vi "Build2DParamArray.vi"(9 "Step Sizes":dbl[](array[numeric]), 10 "Final Values":dbl[](array[numeric]), 11 "Initial Values":dbl[](array[numeric])) -> (2 "Parameter Array":dbl[][](array[numeric]))   [LabVIEW 2013]
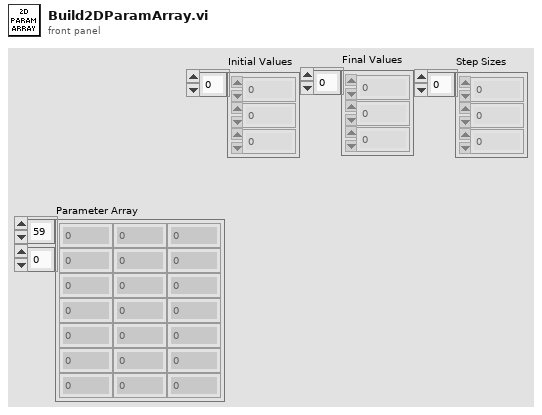
[diagram p1: front panel]
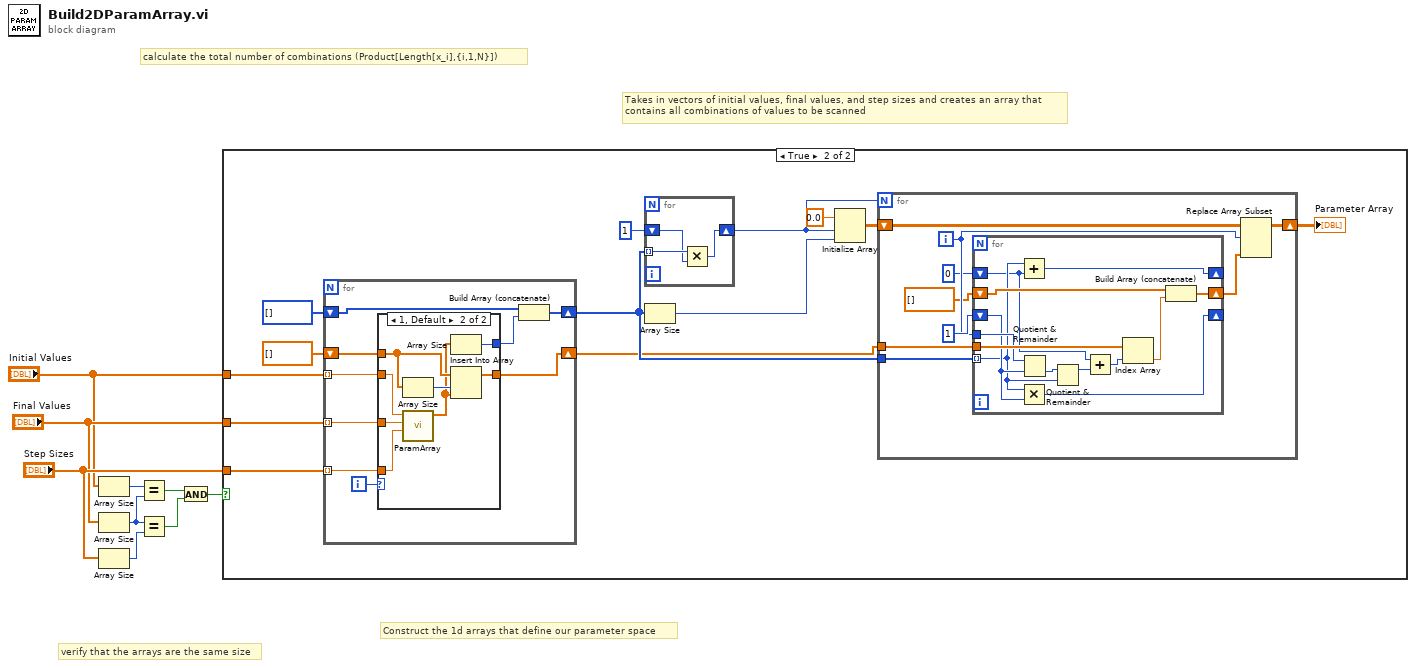
[diagram p0: block diagram]
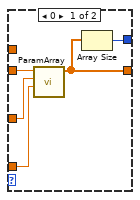
[diagram p3: hidden frame]
diagram:
  # "calculate the total number of combinations (Product[Length[x_i],{i,1,N}])"
  # "Construct the 1d arrays that define our parameter space"
  # "Takes in vectors of initial values, final values, and step sizes and creates an array that\ncontains all combinations of values to be scanned"
  # "verify that the arrays are the same size"
  n1 = Array Size(array="Initial Values") -> (size(s)=w7:i32)
  n2 = Array Size(array="Final Values") -> (size(s)=w8:i32)
  n3 = Array Size(array="Step Sizes") -> (size(s)=w9:i32)
  n4 = Equal?(x=w7, y=w8) -> (x = y?=w6:bool)
  n5 = Equal?(x=w8, y=w9) -> (x = y?=w5:bool)
  n6 = And(x=w6, y=w5) -> (x .and. y?=w4:bool)
  n7 = case shown="True" w4 {
    tunnel: "Step Sizes" -> [_ w22]
    tunnel: "Final Values" -> [_ w21]
    tunnel: "Initial Values" -> [_ w20]
    frame False {
    }
    frame True {
      n8 = for {
        tunnel: w22 -> [w56] mode=indexing
        tunnel: w21 -> [w55] mode=indexing
        tunnel: w20 -> [w54] mode=indexing
        shift-right: [w49] -> w13
        shift-left: dbl[] [] ("Array") -> [w48]
        shift-right: [w51] -> w14
        shift-left: i32[] [] -> [w52]
        i -> [w50]
        n9 = case shown="1, Default" w50 {
          tunnel: w56 -> [w61 w67]
          tunnel: w55 -> [w60 w68]
          tunnel: w54 -> [w59 w69]
          tunnel: [w57 w64] -> w49
          tunnel: [w58 w62] -> w53
          tunnel: w48 -> [_ w66]
          frame 0 {
            n10 = call "ParamArray.vi"("Step Size"=w61, "Final Value"=w60, "Initial Value"=w59) -> ("Array"=w57:dbl[])  [unwired: 8 in]
            n11 = Array Size(array=w57) -> (size(s)=w58:i32)
          }
          frame 1, Default {
            n12 = Array Size(array=w66) -> (size(s)=w65:i32)
            n13 = call "ParamArray.vi"("Step Size"=w67, "Final Value"=w68, "Initial Value"=w69) -> ("Array"=w63:dbl[])  [unwired: 8 in]
            n14 = Array Size(array=w63) -> (size(s)=w62:i32)
            n15 = Insert Into Array(array=w66, index=w65, new element=w63) -> (w64:dbl[])
          }
        }
        n16 = Build Array (concatenate)(w52, w53) -> (w51:i32[])
      }
      n17 = for {
        tunnel: w14 -> [w47] mode=indexing
        shift-right: [w46] -> w16
        shift-left: 1 -> [w45]
        n18 = Multiply(x=w47, y=w45) -> (x*y=w46:i32)
      }
      n19 = Array Size(array=w14) -> (size(s)=w19:i32)
      n20 = Initialize Array(0.0 ("element"), w16, w19) -> (w15:dbl[][])
      n21 = for {
        N: w16 -> [_]
        shift-right: [w30] -> w10
        shift-left: w15 -> [w31]
        tunnel: w14 -> [w29]
        tunnel: w13 -> [w27]
        i -> [w26]
        n22 = for {
          tunnel: w29 -> [w36] mode=indexing
          shift-right: [w44] -> _
          shift-left: 1 -> [w37]
          tunnel: w27 -> [w43]
          tunnel: w26 -> [w42]
          shift-right: [w38] -> w25
          shift-left: dbl[] [] -> [w39]
          shift-right: [w35] -> _
          shift-left: 0 -> [w34]
          n23 = Add(x=w36, y=w34) -> (x+y=w35:i32)
          n24 = Multiply(x=w36, y=w37) -> (x*y=w44:i32)
          n25 = Quotient & Remainder(x=w42, y=w37) -> (floor(x/y)=w41:i32)  [unwired: 1 out]
          n26 = Quotient & Remainder(x=w41, y=w36) -> (x-y*floor(x/y)=w33:i32)  [unwired: 1 out]
          n27 = Add(x=w34, y=w33) -> (x+y=w32:i32)
          n28 = Index Array(array=w43, index=w32) -> (element=w40:dbl)
          n29 = Build Array (concatenate)(w39, w40) -> (w38:dbl[])
        }
        n30 = Replace Array Subset(array=w31, new element=w25, index (row)=w26) -> (w30:dbl[][])  [unwired: 1 in]
      }
      "Parameter Array" <- w10
    }
  }
